vi "Test Server.vi"   [LabVIEW 2012]
uses:
  <vilib>/DAQmx/write.llb/DAQmx Write (Digital 1D Bool NChan 1Samp 1Line).vi
  <vilib>/DAQmx/miscellaneous.llb/DAQmx Fill In Error Info.vi
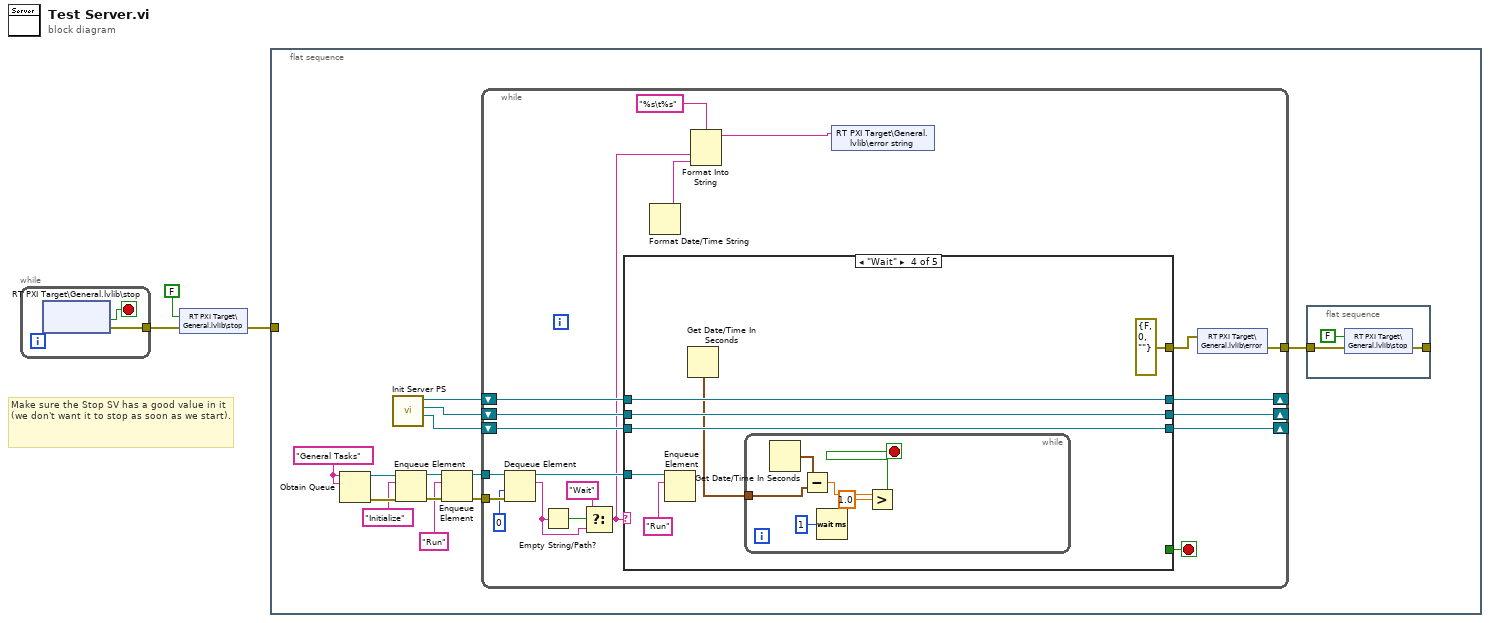
[diagram p0: block diagram]
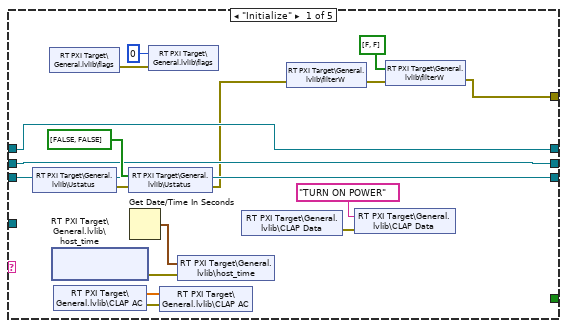
[diagram p2: hidden frame]
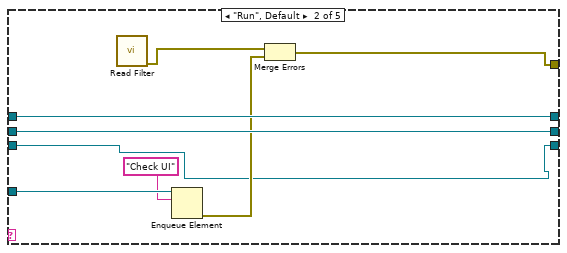
[diagram p3: hidden frame]
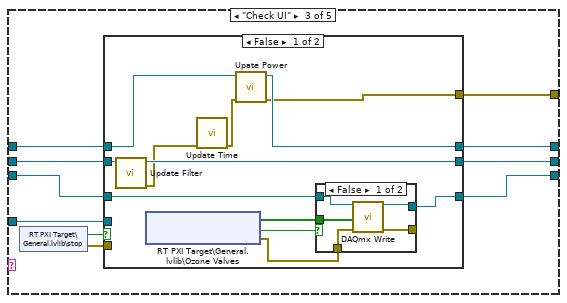
[diagram p4: hidden frame]
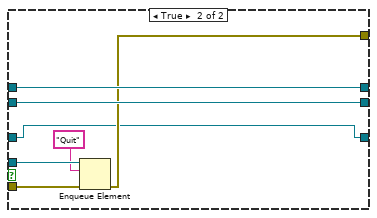
[diagram p6: hidden frame]
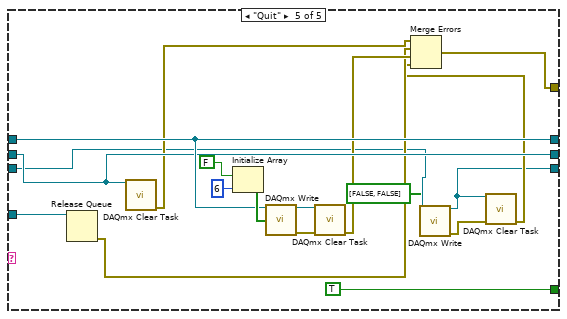
[diagram p7: hidden frame]
diagram:
  # "Make sure the Stop SV has a good value in it (we don't want it to stop as soon as we start)."
  n1 = while {
    tunnel: [w4] -> w2
    stop <- w5 stop-if-true
    n2 = shared-variable "RT PXI Target\\General.lvlib\\stop"() -> (error out=w4:errorcluster, w5:bool)  [unwired: 2 in, 1 out]
  }
  n3 = shared-variable "RT PXI Target\\General.lvlib\\stop"(FALSE ("stop"), error in=w2) -> (error out=w1:errorcluster)
  n4 = flat-sequence {
    tunnel: w1 -> [_]
    frame #0 {
      w17 = "General Tasks" ("name (unnamed)")
      n5 = Obtain Queue(name (unnamed)=w17, element data type=w17) -> (queue out=w16:refnum<queue>, error out=w15:errorcluster)  [unwired: 3 in, 1 out]
      n6 = call "Init Server PS.vi"() -> ("Ozone Out"=w6:refnum<k21>, "Filter Out Task"=w7:refnum<k21>, "PS Switch Out"=w8:refnum<k21>)  [unwired: 8 in, 1 out]
      n7 = Enqueue Element(queue=w16, element="Initialize", error in (no error)=w15) -> (queue out=w13:refnum<queue>, error out=w12:errorcluster)  [unwired: 1 in, 1 out]
      n8 = Enqueue Element(queue=w13, element="Run", error in (no error)=w12) -> (queue out=w10:refnum<queue>, error out=w11:errorcluster)  [unwired: 1 in, 1 out]
      n9 = while {
        tunnel: w11 -> [w33]
        tunnel: w10 -> [w34]
        shift-right: [w35] -> _
        shift-left: w7 -> [w36]
        shift-right: [w37] -> _
        shift-left: w8 -> [w38]
        tunnel: [w25] -> w18
        shift-right: [w24] -> _
        shift-left: w6 -> [w23]
        stop <- w28 stop-if-true
        n10 = Dequeue Element(queue=w34, timeout in ms (-1)=0, error in (no error)=w33) -> (queue out=w29:refnum<queue>, element=w31:string)  [unwired: 2 out]
        n11 = Empty String/Path?(string/path=w31) -> (empty?=w32:bool)
        n12 = Select(t="Wait", s=w32, f=w31) -> (s? t:f=w21:string)
        n13 = case shown="\"Wait\"" w21 {
          tunnel: [w39 w59 w68 errorcluster {"status"=FALSE, "code"=0, "source"=""} ("error IO") w117] -> w26
          tunnel: w38 -> [w43 w61 w71 w105 w124]
          tunnel: [w43 w61 w69 w105 w124] -> w37
          tunnel: w36 -> [w42 w60 w73 w104 w123]
          tunnel: [w42 w60 w72 w104 w123] -> w35
          tunnel: w29 -> [_ w63 w70 w103 w121]
          tunnel: [_ _ _ _ TRUE] -> w28
          tunnel: [w41 w57 w65 w101 w113] -> w24
          tunnel: w23 -> [w41 w57 w64 w101 w116]
          frame "Initialize" {
            n14 = shared-variable "RT PXI Target\\General.lvlib\\Ustatus"() -> (error out=w54:errorcluster)  [unwired: 1 in, 1 out]
            n15 = shared-variable "RT PXI Target\\General.lvlib\\flags"() -> (error out=w51:errorcluster)  [unwired: 1 in, 1 out]
            n16 = shared-variable "RT PXI Target\\General.lvlib\\host_time"() -> (error out=w52:errorcluster)  [unwired: 2 in, 2 out]
            n17 = shared-variable "RT PXI Target\\General.lvlib\\CLAP AC"() -> (w45:sgl[], error out=w46:errorcluster)  [unwired: 1 in]
            n18 = shared-variable "RT PXI Target\\General.lvlib\\Ustatus"(bool[] [FALSE, FALSE], error in=w54) -> (error out=w40:errorcluster)
            n19 = Get Date/Time In Seconds() -> (seconds since 1Jan1904=w53:timestamp)
            n20 = shared-variable "RT PXI Target\\General.lvlib\\flags"(u8 0 ("flags"), error in=w51) -> ()  [unwired: 1 out]
            n21 = shared-variable "RT PXI Target\\General.lvlib\\CLAP AC"(w45, error in=w46) -> ()  [unwired: 1 out]
            n22 = shared-variable "RT PXI Target\\General.lvlib\\host_time"(w53, error in=w52) -> ()  [unwired: 1 out]
            n23 = shared-variable "RT PXI Target\\General.lvlib\\CLAP Data"() -> (error out=w48:errorcluster)  [unwired: 1 in, 1 out]
            n24 = shared-variable "RT PXI Target\\General.lvlib\\filterW"(error in=w40) -> (error out=w50:errorcluster)  [unwired: 1 out]
            n25 = shared-variable "RT PXI Target\\General.lvlib\\CLAP Data"("TURN ON POWER" ("CLAP Data"), error in=w48) -> ()  [unwired: 1 out]
            n26 = shared-variable "RT PXI Target\\General.lvlib\\filterW"(bool[] [FALSE, FALSE] ("filterW"), error in=w50) -> (error out=w39:errorcluster)
          }
          frame "Run", Default {
            n27 = call "Read Filter.vi"() -> ("error out"=w56:errorcluster)  [unwired: 11 in]
            n28 = Enqueue Element(queue=w63, element="Check UI") -> (error out=w58:errorcluster)  [unwired: 2 in, 2 out]
            n29 = Merge Errors(w56, w58) -> (w59:errorcluster)
          }
          frame "Check UI" {
            n30 = shared-variable "RT PXI Target\\General.lvlib\\stop"() -> (w66:bool, error out=w67:errorcluster)  [unwired: 1 in]
            n31 = case shown="False" w66 {
              tunnel: w73 -> [w85 w95]
              tunnel: [w84 w95] -> w72
              tunnel: w71 -> [w83 w96]
              tunnel: w70 -> [_ w98]
              tunnel: [w82 w96] -> w69
              tunnel: [w75 w93] -> w68
              tunnel: w67 -> [_ w94]
              tunnel: [w78 w92] -> w65
              tunnel: w64 -> [w79 w92]
              frame False {
                n32 = call "Update Filter.vi"("Refnum in"=w85) -> ("error out"=w74:errorcluster, "Refnum out"=w84:refnum<k21>)  [unwired: 9 in]
                n33 = shared-variable "RT PXI Target\\General.lvlib\\Ozone Valves"() -> (w77:bool[], error out=w76:errorcluster, w80:bool)  [unwired: 2 in]
                n34 = call "Update Time.vi"("error in"=w74) -> ("error out"=w81:errorcluster)  [unwired: 10 in]
                n35 = call "Upate Power.vi"("error in"=w81, "Refnum in"=w83) -> ("error out"=w75:errorcluster, "Refnum out"=w82:refnum<k21>)  [unwired: 8 in]
                n36 = case shown="False" w80 {
                  tunnel: w79 -> [w90 w91]
                  tunnel: [w89 w91] -> w78
                  tunnel: w77 -> [w88 _]
                  tunnel: w76 -> [w87 _]
                  tunnel: [w86 _] -> _
                  frame False {
                    n37 = call-poly <vilib>:"DAQmx Write.vi"("task/channels in"=w90, "data"=w88, "error in"=w87) -> ("task out"=w89:refnum<k21>, "error out"=w86:errorcluster)  [unwired: 10 in, 1 out]
                  }
                  frame True {
                  }
                }
              }
              frame True {
                n38 = Enqueue Element(queue=w98, element="Quit", error in (no error)=w94) -> (error out=w93:errorcluster)  [unwired: 1 in, 2 out]
              }
            }
          }
          frame "Wait" {
            n39 = Enqueue Element(queue=w103, element="Run") -> ()  [unwired: 2 in, 3 out]
            n40 = Get Date/Time In Seconds() -> (seconds since 1Jan1904=w100:timestamp)
            n41 = while {
              tunnel: w100 -> [w110]
              stop <- w106 stop-if-true
              n42 = Get Date/Time In Seconds() -> (seconds since 1Jan1904=w109:timestamp)
              n43 = Subtract(x=w109, y=w110) -> (x-y=w108:dbl)
              n44 = Wait (ms)(milliseconds to wait=u32 1) -> ()  [unwired: 1 out]
              n45 = Greater?(x=w108, y=1.0) -> (0:w106:bool)
            }
          }
          frame "Quit" {
            n46 = Release Queue(queue=w121) -> (error out=w118:errorcluster)  [unwired: 2 in, 2 out]
            n47 = call <vilib>:"DAQmx Clear Task.vi"("task in"=w123) -> ("error out"=w119:errorcluster)  [unwired: 14 in]
            n48 = Initialize Array(FALSE, 6 ("dimension size")) -> (w127:bool[])
            n49 = call-poly <vilib>:"DAQmx Write.vi"("task/channels in"=w124, "data"=w127) -> ("task out"=w128:refnum<k21>, "error out"=w129:errorcluster)  [unwired: 11 in, 1 out]
            n50 = call <vilib>:"DAQmx Clear Task.vi"("task in"=w128, "error in"=w129) -> ("error out"=w120:errorcluster)  [unwired: 13 in]
            n51 = call-poly <vilib>:"DAQmx Write.vi"("task/channels in"=w116, "data"=bool[] [FALSE, FALSE]) -> ("task out"=w113:refnum<k21>, "error out"=w115:errorcluster)  [unwired: 11 in, 1 out]
            n52 = call <vilib>:"DAQmx Clear Task.vi"("task in"=w113, "error in"=w115) -> ("error out"=w114:errorcluster)  [unwired: 13 in]
            n53 = Merge Errors(w119, w118, w120, w114) -> (w117:errorcluster)
          }
        }
        n54 = Format Date/Time String() -> (date/time string=w20:string)  [unwired: 3 in]
        n55 = Format Into String(format string="%s\t%s", w21, w20) -> (resulting string=w19:string)  [unwired: 2 in, 1 out]
        n56 = shared-variable "RT PXI Target\\General.lvlib\\error string"(w19) -> ()  [unwired: 1 in, 1 out]
        n57 = shared-variable "RT PXI Target\\General.lvlib\\error"(w26) -> (error out=w25:errorcluster)  [unwired: 1 in]
      }
      n58 = flat-sequence {
        tunnel: w18 -> [w131]
        tunnel: [w130] -> _
        frame #0 {
          n59 = shared-variable "RT PXI Target\\General.lvlib\\stop"(FALSE ("stop"), error in=w131) -> (error out=w130:errorcluster)
        }
      }
    }
  }
